vi "Aggregate Scan.vi"(6 "Local Data":T2, 8 "error in":errorcluster) -> (0 "error out":errorcluster, 2 "Acquisition Scan":T1 {"Time Stamp" format="%<%x %.3X>T"}, 4 "Local Data Out":T2)   [LabVIEW 2025]
uses:
  Controls/Local Data_Acquisition.ctl
  Controls/Acquisition Packet.ctl
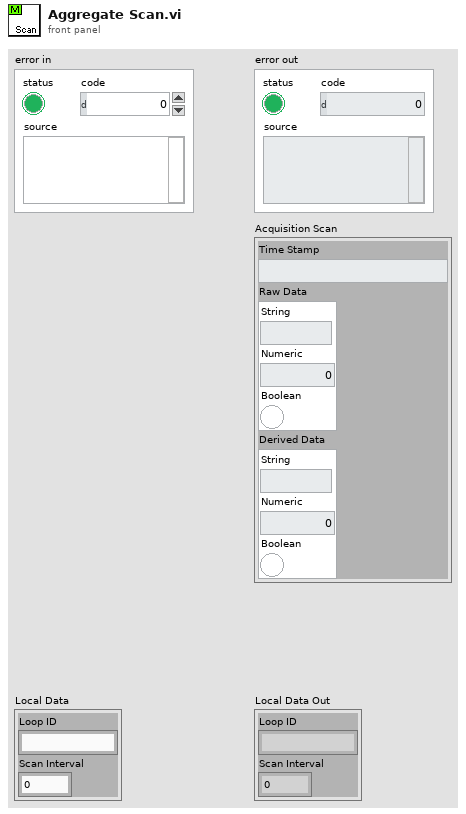
[diagram p1: front panel]
types:
  T1 = typedef "Acquisition Packet.ctl" = cluster{"Time Stamp":timestamp, "Raw Data":cluster{"String":string, "Numeric":dbl, "Boolean":bool}, "Derived Data":cluster{"String":string, "Numeric":dbl, "Boolean":bool}}
  T2 = typedef "Local Data_Acquisition.ctl" = cluster{"Loop ID":string, "Scan Interval":u32}
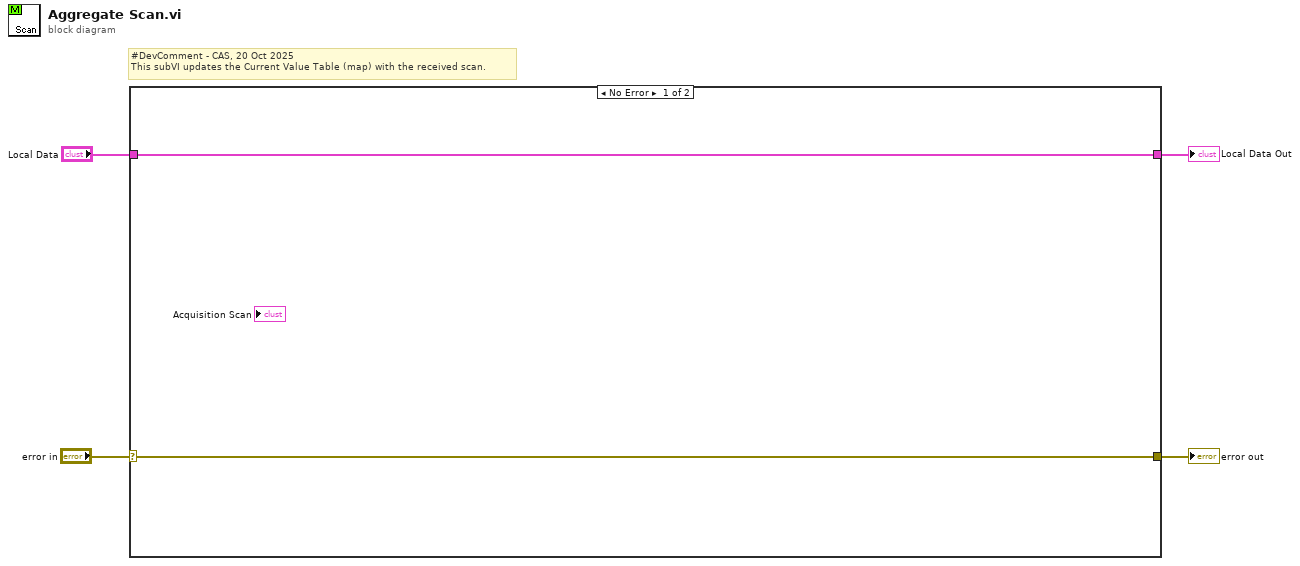
[diagram p0: block diagram]
diagram:
  # "#DevComment - CAS, 20 Oct 2025\nThis subVI updates the Current Value Table (map) with the received scan."
  n1 = case shown="No Error" "error in" {
    selector: "error in" -> [w6 w8]
    tunnel: [w6 w8] -> w3
    tunnel: [w5 w7] -> w2
    tunnel: "Local Data" -> [w5 w7]
    frame No Error {
    }
    frame Error {
    }
  }
  "error out" <- w3
  "Local Data Out" <- w2
